vi "AFM_DLog.GetPublicEvents.vi"(8 "error in (no error)":errorcluster, 11 "Instrument.AFM_DLog in":refnum<class "Instrument.AFM_DLog.lvclass">) -> (0 "error out":errorcluster, 2 "Public Events":T1, 3 "Instrument.AFM_DLog out":refnum<class "Instrument.AFM_DLog.lvclass">)   [LabVIEW 2019, in "Instrument.AFM_DLog.lvclass"]
uses:
  Instrument.AFM_DLog.lvclass
  <userlib>/LevyLab/RemoteControl/RemoteControl/Typedefs/Message--Cluster.ctl
  <userlib>/LevyLab/RemoteControl/RemoteControl/RemoteControl.lvclass
  Typedefs/PublicEvents--AFM_DLog.MessageFromProcess.ctl
  Typedefs/PublicEvents--Cluster.ctl
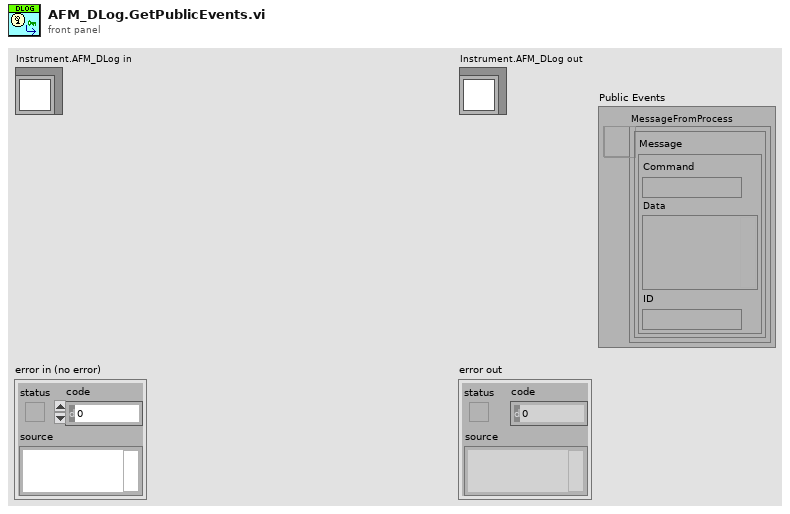
[diagram p1: front panel]
types:
  T1 = typedef "Instrument.AFM_DLog.lvclass/PublicEvents--Cluster.ctl" = cluster{"MessageFromProcess":refnum<user-event>}
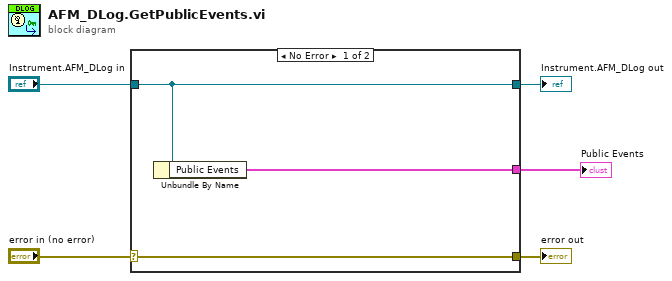
[diagram p0: block diagram]
diagram:
  n1 = case shown="No Error" "error in (no error)" {
    selector: "error in (no error)" -> [w8 w9]
    tunnel: [w8 w9] -> w4
    tunnel: [w7 w10] -> w2
    tunnel: "Instrument.AFM_DLog in" -> [w7 w10]
    tunnel: [w6 _] -> w1
    frame No Error {
      n2 = Unbundle By Name(w7) -> ("Public Events"=w6:T1)
    }
    frame Error {
    }
  }
  "error out" <- w4
  "Instrument.AFM_DLog out" <- w2
  "Public Events" <- w1
